vi "AVTCP-Build.vi"() -> ()   [LabVIEW 2020]
uses:
  <vilib>/AppBuilder/AB_API_Simple/Build (path).vi
  <vilib>/AppBuilder/AB_API_Simple/NI_App_Builder_API.lvlib
panel:
  out "Status":string
  in  "Version":T1={"Major"=3, "Minor"=0, "Fix"=0, "Build"=0}
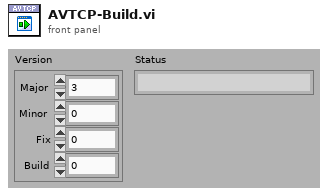
[diagram p1: front panel]
types:
  T1 = cluster{"Major":i32, "Minor":i32, "Fix":i32, "Build":i32}
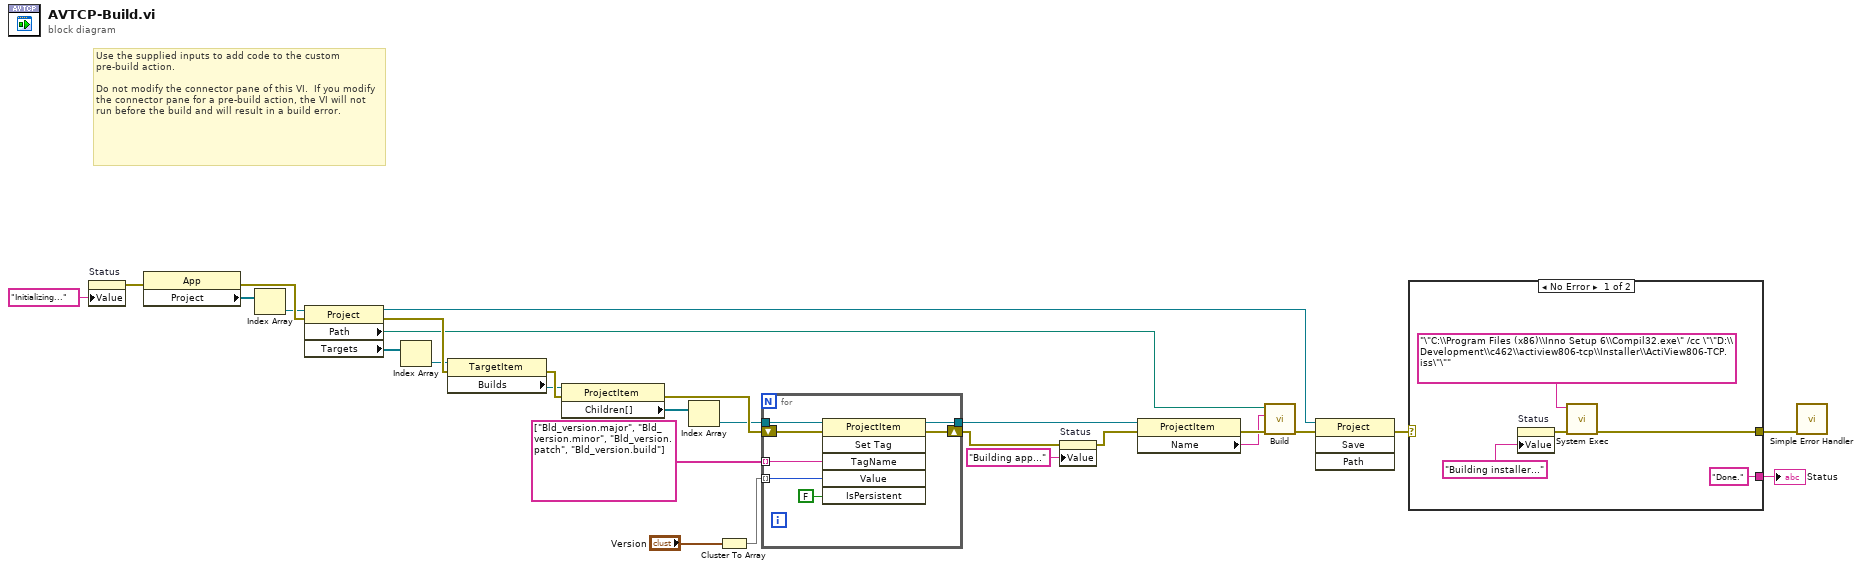
[diagram p0: block diagram]
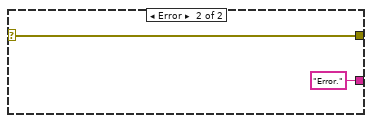
[diagram p2: hidden frame]
diagram:
  # "Use the supplied inputs to add code to the custom pre-build action.\n\nDo not modify the connector pane of this VI.  If you modify the connector pane for a pre-build action, the VI will not run before the build and will result in a build error."
  n1 = property on="Status" class="Str"("Value"="Initializing..." ("Status")) -> (error out=w8:errorcluster)  [unwired: 2 in, 1 out]
  n2 = property class="App"(error in=w8) -> (error out=w28:errorcluster, "Project"=w25:refnum<vi>[])  [unwired: 1 in, 1 out]
  n3 = Index Array(array=w25) -> (element=w24:refnum<vi>)  [unwired: 1 in]
  n4 = property class="Project"(reference=w24, error in=w28) -> (reference out=w19:refnum<vi>, error out=w27:errorcluster, "Path"=w12:path, "Targets"=w10:refnum<vi>[])
  n5 = Index Array(array=w10) -> (element=w23:refnum<vi>)  [unwired: 1 in]
  n6 = property class="TargetItem"(reference=w23, error in=w27) -> (error out=w26:errorcluster, "Builds"=w22:refnum<vi>)  [unwired: 1 out]
  n7 = property class="ProjectItem"(reference=w22, error in=w26) -> (error out=w21:errorcluster, "Children[]"=w20:refnum<vi>[])  [unwired: 1 out]
  n8 = Index Array(array=w20) -> (element=w16:refnum<vi>)  [unwired: 1 in]
  n9 = Cluster To Array(cluster="Version") -> (array=w17:i32[])
  n10 = for {
    tunnel: w16 -> [w34]
    tunnel: w17 -> [w32] mode=indexing
    shift-right: [w30] -> w6
    shift-left: w21 -> [w33]
    tunnel: string[] ["Bld_version.major", "Bld_version.minor", "Bld_version.patch", "Bld_version.build"] -> [w31] mode=indexing
    tunnel: [w29] -> w15
    n11 = invoke class="ProjectItem" method="Set Tag"(reference=w34, error in=w33, "TagName"=w31, "Value"=w32, "IsPersistent"=FALSE ("Is Persistent")) -> (reference out=w29:refnum<vi>, error out=w30:errorcluster)  [unwired: 1 in, 4 out]
  }
  n12 = property on="Status" class="Str"(error in=w6, "Value"="Building app..." ("Status")) -> (error out=w5:errorcluster)  [unwired: 1 in, 1 out]
  n13 = property class="ProjectItem"(reference=w15, error in=w5) -> (error out=w14:errorcluster, "Name"=w13:string)  [unwired: 1 out]
  n14 = call-poly <vilib>:"Build.vi"("error in (no error)"=w14, "Name of build specification (if empty: build all)"=w13, "Path to project"=w12) -> ("error out"=w11:errorcluster)  [unwired: 7 in, 1 out]
  n15 = invoke class="Project" method="Save"(reference=w19, error in=w11) -> (error out=w1:errorcluster)  [unwired: 2 in, 3 out]
  n16 = case shown="No Error" w1 {
    selector: w1 -> [_ w42]
    tunnel: [w39 w42] -> w9
    tunnel: ["Done." "Error."] -> w3
    frame No Error {
      n17 = property on="Status" class="Str"("Value"="Building installer..." ("Status")) -> (error out=w38:errorcluster)  [unwired: 2 in, 1 out]
      n18 = call <vilib>:"System Exec.vi"("error in (no error)"=w38, "command line"="\"C:\\Program Files (x86)\\Inno Setup 6\\Compil32.exe\" /cc \"\"D:\\Development\\c462\\actiview806-tcp\\Installer\\ActiView806-TCP.iss\"\"") -> ("error out"=w39:errorcluster)  [unwired: 6 in, 3 out]
    }
    frame Error {
    }
  }
  "Status" <- w3
  n19 = call <vilib>:"Simple Error Handler.vi"("error in (no error)"=w9) -> ()  [unwired: 4 in, 5 out]
